vi "ConfigUI.vi"(8 "error in":errorcluster) -> (0 "error out":errorcluster)   [LabVIEW 2011]
uses:
  SubVIs/Controls/Control FP Objects - Operations.ctl
  SubVIs/Controls/INIT- READ - WRITE.ctl
  SubVIs/Controls/Init-Write-Read.ctl
  SubVIs/Controls/GetModueDescriptionsOperations.ctl
  SubVIs/Controls/Config UI Global Stop - Operations.ctl
  SubVIs/Controls/TransparencyEffectOperations.ctl
  SubVIs/Controls/ModulePicCluster.ctl
panel:
  in  "Stop":bool
  in  "Ready":bool
  in  "Testpanel":bool
  in  "Tab":enum32{"STATUS OK", "NO CHASSIS"}(tab)
  out "Info":string
  in  "BubbleTabs":T1(tab)
  in  "Slot BTN 8":bool
  in  "Slot BTN 7":bool
  in  "Slot BTN 6":bool
  in  "Slot BTN 5":bool
  in  "Slot BTN 4":bool
  in  "Slot BTN 3":bool
  in  "Slot BTN 2":bool
  in  "Slot BTN 1":bool
  out "ModSTR 8":string
  out "ModSTR 7":string
  out "ModSTR 6":string
  out "ModSTR 5":string
  out "ModSTR 4":string
  out "ModSTR 3":string
  out "ModSTR 2":string
  out "ModSTR 1":string
  out "Slot 8":picture
  out "Slot 7":picture
  out "Slot 6":picture
  out "Slot 5":picture
  out "Slot 4":picture
  out "Slot 3":picture
  out "Slot 2":picture
  out "Slot 1":picture
  out "CHASSIS_PIC":picture
  # "Configure your system by Clicking the modules"
  # "No CompactDAQ Chassis found! Please Connect your CompactDAQ Device or create simulated device in MAX!"
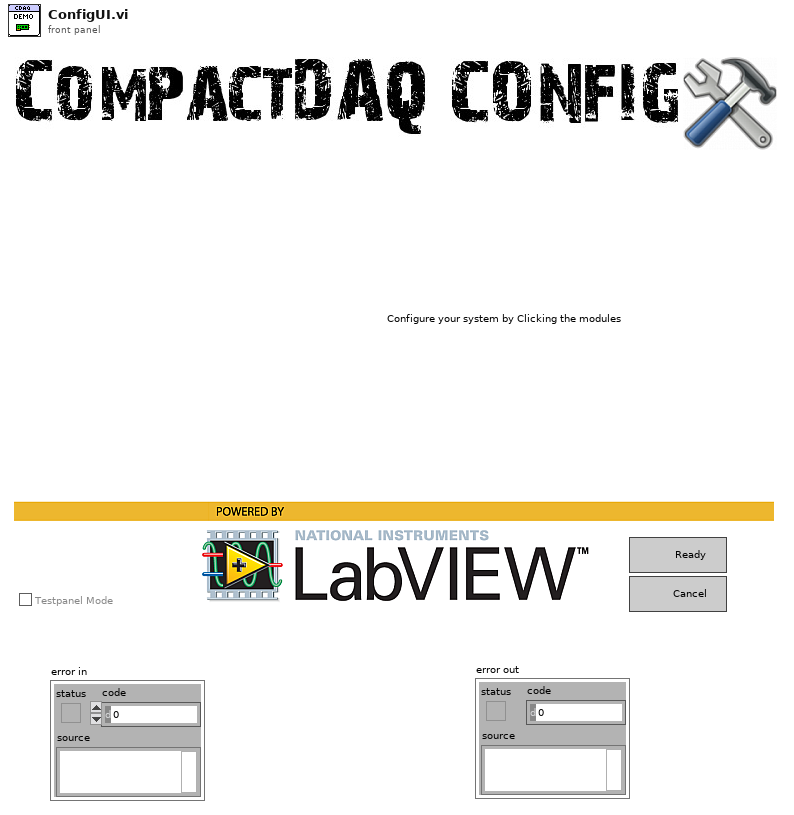
[diagram p1: front panel]
types:
  T1 = enum32{"Bubble1", "Bubble2", "Bubble3", "Bubble4", "Bubble5", "Bubble6", "Bubble7", "Bubble8", "EMPTY"}
  T2 = typedef "Control FP Objects - Operations.ctl" = enum16{"INIT", "CHANGE CHASSIS", "END"}
  T3 = typedef "INIT- READ - WRITE.ctl" = enum16{"INIT", "READ", "WRITE"}
  T4 = typedef "Init-Write-Read.ctl" = enum16{"INIT", "WRITE", "READ", "READ ALL"}
  T5 = typedef "GetModueDescriptionsOperations.ctl" = enum16{"INIT", "GET"}
  T6 = typedef "Config UI Global Stop - Operations.ctl" = enum16{"INIT", "STATUS", "STOP"}
  T7 = typedef "TransparencyEffectOperations.ctl" = enum16{"Show", "Hide 80%", "Hide All"}
  T8 = typedef "ModulePicCluster.ctl" = cluster{"Slot Nr":i32, "ModulePic":picture}
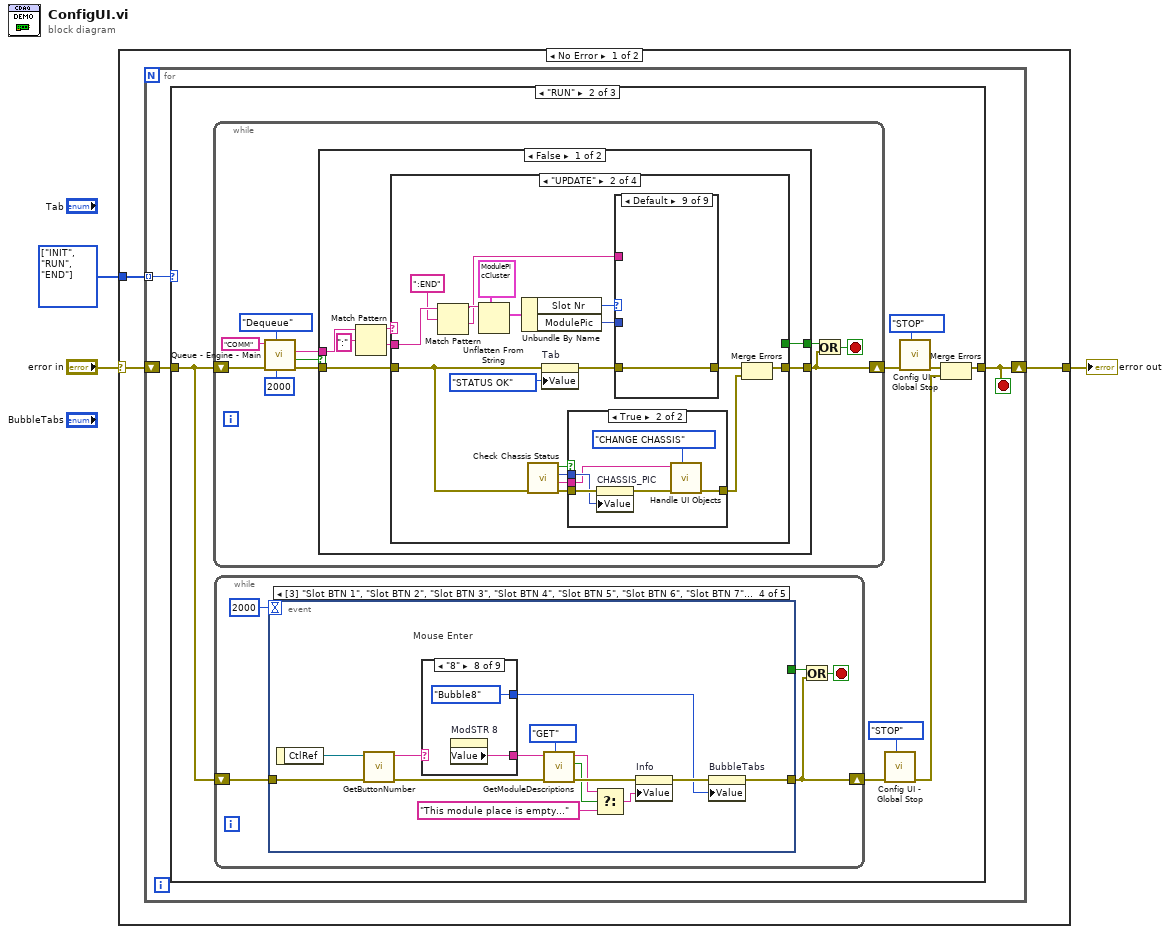
[diagram p0: block diagram]
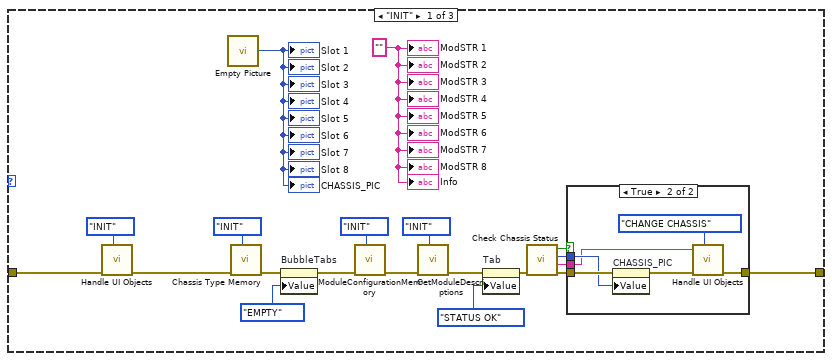
[diagram p2: hidden frame]
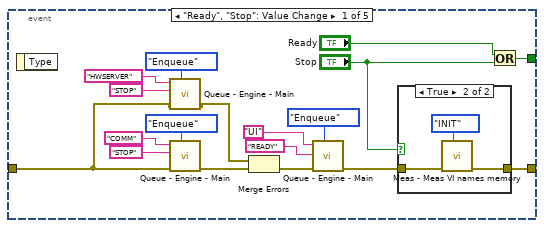
[diagram p4: hidden frame]
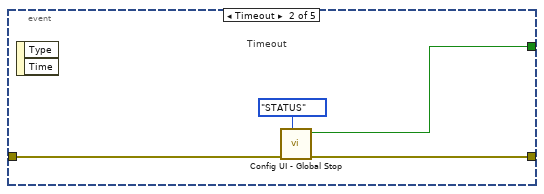
[diagram p6: hidden frame]
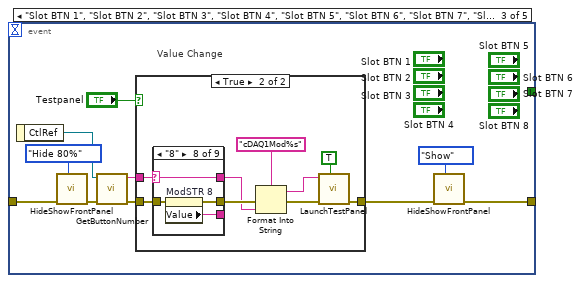
[diagram p7: hidden frame]
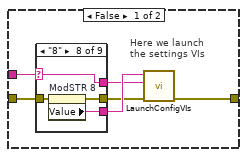
[diagram p8: hidden frame]
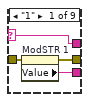
[diagram p9: hidden frame]
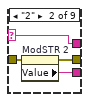
[diagram p10: hidden frame]
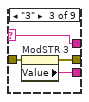
[diagram p11: hidden frame]
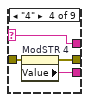
[diagram p12: hidden frame]
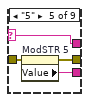
[diagram p13: hidden frame]
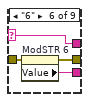
[diagram p14: hidden frame]
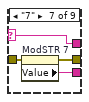
[diagram p15: hidden frame]
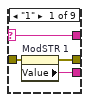
[diagram p17: hidden frame]
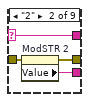
[diagram p18: hidden frame]
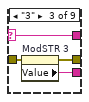
[diagram p19: hidden frame]
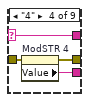
[diagram p20: hidden frame]
diagram:
  w3 = enum16{"INIT", "RUN", "END"}[] [enum."INIT", enum."RUN", enum."END"] items=["INIT", "RUN", "END"]
  n1 = case shown="No Error" "error in" {
    selector: "error in" -> [w4 w307]
    tunnel: w3 -> [w6 _]
    tunnel: [w5 w307] -> w2
    frame No Error {
      n2 = for {
        tunnel: w6 -> [w9] mode=indexing
        shift-right: [w7] -> w5
        shift-left: w4 -> [w8]
        stop <- w7 stop-if-true
        n3 = case shown="\"RUN\"" w9 {
          tunnel: [w18 w44 w303] -> w7
          tunnel: w8 -> [w13 w43 w306]
          frame "INIT" {
            w29 = "" ("ModSTR 1")
            n4 = call "Handle UI Objects.vi"("Operation"=Control_FP_Objects_-_Operations."INIT", "error in"=w13) -> ("error out"=w12:errorcluster)  [unwired: 9 in]
            n5 = call "Empty Picture"() -> ("empty picture"=→"Slot 1" →"Slot 2" →"Slot 3" →"Slot 4" →"Slot 5" →"Slot 6" →"Slot 7" →"Slot 8" →"CHASSIS_PIC":picture)
            n6 = call "Chassis Type Memory.vi"("Operation"=INIT-_READ_-_WRITE."INIT", "Error In"=w12) -> ("Error Out"=w15:errorcluster)  [unwired: 8 in, 1 out]
            n7 = property on="BubbleTabs" class="TabCtl (strict)"(error in=w15, "Value"=T1."EMPTY" ("BubbleTabs")) -> (error out=w14:errorcluster)  [unwired: 1 in, 1 out]
            n8 = call "ModuleConfigurationMemory.vi"("Operation"=Init-Write-Read."INIT", "Error In"=w14) -> ("Error Out"=w26:errorcluster)  [unwired: 5 in, 4 out]
            n9 = call "GetModuleDescriptions.vi"("Operation"=GetModueDescriptionsOperations."INIT", "Error In"=w26) -> ("Error Out"=w24:errorcluster)  [unwired: 7 in, 2 out]
            n10 = property on="Tab" class="TabCtl (strict)"(error in=w24, "Value"=enum32{"STATUS OK", "NO CHASSIS"}."STATUS OK" ("Tab")) -> (error out=w17:errorcluster)  [unwired: 1 in, 1 out]
            n11 = call "Check Chassis Status.vi"("error in (no error)"=w17) -> ("error out"=w21:errorcluster, "Chassis type Out"=w10:string, "Chassis Pic Out"=w20:picture, "Update?"=w19:bool)  [unwired: 7 in]
            n12 = case shown="True" w19 {
              tunnel: w21 -> [w30 w36]
              tunnel: [w30 w34] -> w18
              tunnel: w20 -> [_ w35]
              tunnel: w10 -> [_ w31]
              frame False {
                # "nothing to update"
              }
              frame True {
                n13 = property on="CHASSIS_PIC" class="Pict"(error in=w36, "Value"=w35) -> (error out=w33:errorcluster)  [unwired: 1 in, 1 out]
                n14 = call "Handle UI Objects.vi"("Operation"=Control_FP_Objects_-_Operations."CHANGE CHASSIS", "error in"=w33, "String In"=w31) -> ("error out"=w34:errorcluster)  [unwired: 8 in]
              }
            }
            "ModSTR 1" <- w29
            "ModSTR 2" <- w29
            "ModSTR 3" <- w29
            "ModSTR 4" <- w29
            "ModSTR 5" <- w29
            "ModSTR 7" <- w29
            "ModSTR 8" <- w29
            "ModSTR 6" <- w29
            "Info" <- w29
          }
          frame "RUN" {
            n15 = while {
              shift-right: [w214] -> w38
              shift-left: w43 -> [w208]
              stop <- w212 stop-if-true
              n16 = call "Queue - Engine - Main.vi"("timeout in ms (-1)"=2000, "Operation"=enum16{"Enqueue", "Dequeue", "Flush", "Release"}."Dequeue", "error in"=w208, "Queue Name In"="COMM" ("name (unnamed)")) -> ("error out"=w207:errorcluster, "timed out?"=w206:bool, "Data Out"=w205:string)  [unwired: 5 in]
              n17 = case shown="False" w206 {
                tunnel: w207 -> [w221 w290]
                tunnel: [w220 w288] -> w214
                tunnel: w205 -> [w218 _]
                tunnel: [w215 w287] -> w213
                frame False {
                  n18 = Match Pattern(string=w218, regular expression=":") -> (before substring=w219:string, after substring=w216:string)  [unwired: 1 in, 2 out]
                  n19 = case shown="\"UPDATE\"" w219 {
                    tunnel: w221 -> [w222 w230 w283 w285]
                    tunnel: [w222 w228 w282 w285] -> w220
                    tunnel: w216 -> [_ w234 _ _]
                    tunnel: [_ _ _ TRUE] -> w215
                    frame Default {
                    }
                    frame "UPDATE" {
                      n20 = Match Pattern(string=w234, regular expression=":END") -> (before substring=w236:string, after substring=w235:string)  [unwired: 1 in, 2 out]
                      n21 = Unflatten From String(type=T8 {"Slot Nr"=0, "ModulePic"=bytes[0]}, binary string=w236) -> (value=w239:T8)  [unwired: 3 in, 2 out]
                      n22 = Unbundle By Name(w239) -> ("Slot Nr"=w238:i32, "ModulePic"=w237:picture)
                      n23 = call "Check Chassis Status.vi"("error in (no error)"=w230) -> ("error out"=w227:errorcluster, "Chassis type Out"=w223:string, "Chassis Pic Out"=w225:picture, "Update?"=w224:bool)  [unwired: 7 in]
                      n24 = property on="Tab" class="TabCtl (strict)"(error in=w230, "Value"=enum32{"STATUS OK", "NO CHASSIS"}."STATUS OK" ("Tab")) -> (error out=w231:errorcluster)  [unwired: 1 in, 1 out]
                      n25 = case shown="True" w224 {
                        tunnel: w227 -> [w241 w247]
                        tunnel: [w241 w244] -> w226
                        tunnel: w225 -> [_ w246]
                        tunnel: w223 -> [_ w242]
                        frame False {
                          # "No update"
                        }
                        frame True {
                          n26 = property on="CHASSIS_PIC" class="Pict"(error in=w247, "Value"=w246) -> (error out=w245:errorcluster)  [unwired: 1 in, 1 out]
                          n27 = call "Handle UI Objects.vi"("Operation"=Control_FP_Objects_-_Operations."CHANGE CHASSIS", "error in"=w245, "String In"=w242) -> ("error out"=w244:errorcluster)  [unwired: 8 in]
                        }
                      }
                      n28 = case shown="Default" w238 {
                        tunnel: w237 -> [w249 w253 w257 w263 w267 w271 w275 w277 _]
                        tunnel: w231 -> [w251 w255 w259 w262 w266 w270 w274 w279 w280]
                        tunnel: [w250 w254 w258 w261 w265 w269 w273 w278 w280] -> w229
                        tunnel: w235 -> [w248 w252 w256 w260 w264 w268 w272 w276 _]
                        frame 1 {
                          n29 = property on="ModSTR 1" class="Str"("Value"=w248) -> ()  [unwired: 2 in, 2 out]
                          n30 = property on="Slot 1" class="Pict"(error in=w251, "Value"=w249) -> (error out=w250:errorcluster)  [unwired: 1 in, 1 out]
                        }
                        frame 2 {
                          n31 = property on="ModSTR 2" class="Str"("Value"=w252) -> ()  [unwired: 2 in, 2 out]
                          n32 = property on="Slot 2" class="Pict"(error in=w255, "Value"=w253) -> (error out=w254:errorcluster)  [unwired: 1 in, 1 out]
                        }
                        frame 3 {
                          n33 = property on="ModSTR 3" class="Str"("Value"=w256) -> ()  [unwired: 2 in, 2 out]
                          n34 = property on="Slot 3" class="Pict"(error in=w259, "Value"=w257) -> (error out=w258:errorcluster)  [unwired: 1 in, 1 out]
                        }
                        frame 4 {
                          n35 = property on="ModSTR 4" class="Str"("Value"=w260) -> ()  [unwired: 2 in, 2 out]
                          n36 = property on="Slot 4" class="Pict"(error in=w262, "Value"=w263) -> (error out=w261:errorcluster)  [unwired: 1 in, 1 out]
                        }
                        frame 5 {
                          n37 = property on="ModSTR 5" class="Str"("Value"=w264) -> ()  [unwired: 2 in, 2 out]
                          n38 = property on="Slot 5" class="Pict"(error in=w266, "Value"=w267) -> (error out=w265:errorcluster)  [unwired: 1 in, 1 out]
                        }
                        frame 6 {
                          n39 = property on="ModSTR 6" class="Str"("Value"=w268) -> ()  [unwired: 2 in, 2 out]
                          n40 = property on="Slot 6" class="Pict"(error in=w270, "Value"=w271) -> (error out=w269:errorcluster)  [unwired: 1 in, 1 out]
                        }
                        frame 7 {
                          n41 = property on="ModSTR 7" class="Str"("Value"=w272) -> ()  [unwired: 2 in, 2 out]
                          n42 = property on="Slot 7" class="Pict"(error in=w274, "Value"=w275) -> (error out=w273:errorcluster)  [unwired: 1 in, 1 out]
                        }
                        frame 8 {
                          n43 = property on="ModSTR 8" class="Str"("Value"=w276) -> ()  [unwired: 2 in, 2 out]
                          n44 = property on="Slot 8" class="Pict"(error in=w279, "Value"=w277) -> (error out=w278:errorcluster)  [unwired: 1 in, 1 out]
                        }
                        frame Default {
                        }
                      }
                      n45 = Merge Errors(w229, w226) -> (w228:errorcluster)
                    }
                    frame "NO CHASSIS" {
                      n46 = property on="Tab" class="TabCtl (strict)"(error in=w283, "Value"=enum32{"STATUS OK", "NO CHASSIS"}."NO CHASSIS" ("Tab")) -> (error out=w282:errorcluster)  [unwired: 1 in, 1 out]
                    }
                    frame "STOP" {
                    }
                  }
                }
                frame True {
                  # "Timeout"
                  n47 = call "Check Chassis Status.vi"("error in (no error)"=w290) -> ("error out"=w294:errorcluster, "Chassis type Out"=w291:string, "Chassis Pic Out"=w293:picture, "Update?"=w292:bool)  [unwired: 7 in]
                  n48 = case shown="True" w292 {
                    tunnel: w294 -> [w295 w301]
                    tunnel: [w295 w298] -> w289
                    tunnel: w293 -> [_ w300]
                    tunnel: w291 -> [_ w297]
                    frame False {
                    }
                    frame True {
                      n49 = property on="CHASSIS_PIC" class="Pict"(error in=w301, "Value"=w300) -> (error out=w299:errorcluster)  [unwired: 1 in, 1 out]
                      n50 = call "Handle UI Objects.vi"("Operation"=Control_FP_Objects_-_Operations."CHANGE CHASSIS", "error in"=w299, "String In"=w297) -> ("error out"=w298:errorcluster)  [unwired: 8 in]
                    }
                  }
                  n51 = call "Config UI - Global Stop.vi"("Operation"=Config_UI_Global_Stop_-_Operations."STATUS", "error in (no error)"=w289) -> ("error out"=w288:errorcluster, "Stop?"=w287:bool)  [unwired: 8 in]
                }
              }
              n52 = Or(x=w213, y=w214) -> (x .or. y?=w212:bool)
            }
            n53 = while {
              shift-right: [w48] -> w42
              shift-left: w43 -> [w49]
              stop <- w46 stop-if-true
              n54 = event shown="[3] \"Slot BTN 1\", \"Slot BTN 2\", \"Slot BTN 3\", \"Slot BTN 4\", \"Slot BTN 5\", \"Slot BTN 6\", \"Slot BTN 7\", \"Slot BTN 8\": Mouse Enter" {
                selector: _ -> [_ _ _ _ _]
                dyn-events: _ -> [_ _ _ _ _]
                timeout: 2000 -> [_ _ _ _ _]
                tunnel: [w53 w74 _ _ _] -> w47
                tunnel: [w50 w72 w78 w174 w201] -> w48
                tunnel: w49 -> [w60 w73 w81 w181 w203]
                event "Ready", "Stop": Value Change {
                  n55 = event-data() -> ()  [unwired: 1 in, 1 out]
                  n56 = call "Queue - Engine - Main.vi"("Operation"=enum16{"Enqueue", "Dequeue", "Flush", "Release"}."Enqueue", "error in"=w60, "Queue Data In"="STOP" ("element"), "Queue Name In"="HWSERVER" ("name (unnamed)")) -> ("error out"=w59:errorcluster)  [unwired: 5 in, 2 out]
                  n57 = call "Queue - Engine - Main.vi"("Operation"=enum16{"Enqueue", "Dequeue", "Flush", "Release"}."Enqueue", "error in"=w60, "Queue Data In"="STOP" ("element"), "Queue Name In"="COMM" ("name (unnamed)")) -> ("error out"=w65:errorcluster)  [unwired: 5 in, 2 out]
                  n58 = Merge Errors(w59, w65) -> (w55:errorcluster)
                  n59 = call "Queue - Engine - Main.vi"("Operation"=enum16{"Enqueue", "Dequeue", "Flush", "Release"}."Enqueue", "error in"=w55, "Queue Data In"="READY" ("Queue Name In"), "Queue Name In"="UI") -> ("error out"=w51:errorcluster)  [unwired: 5 in, 2 out]
                  n60 = case shown="True" "Stop" {
                    tunnel: w51 -> [w68 w69]
                    tunnel: [w68 w70] -> w50
                    frame False {
                    }
                    frame True {
                      n61 = call "Meas - Meas VI names memory.vi"("Operation"=INIT-_READ_-_WRITE."INIT", "Error In"=w69) -> ("Error Out"=w70:errorcluster)  [unwired: 8 in, 1 out]
                    }
                  }
                  n62 = Or(x="Ready", y="Stop") -> (x .or. y?=w53:bool)
                }
                event Timeout {
                  # "Timeout"
                  n63 = event-data() -> ()  [unwired: 1 in, 2 out]
                  n64 = call "Config UI - Global Stop.vi"("Operation"=Config_UI_Global_Stop_-_Operations."STATUS", "error in (no error)"=w73) -> ("error out"=w72:errorcluster, "Stop?"=w74:bool)  [unwired: 8 in]
                }
                event "Slot BTN 1", "Slot BTN 2", "Slot BTN 3", "Slot BTN 4", "Slot BTN 5", "Slot BTN 6", "Slot BTN 7", "Slot BTN 8": Value Change {
                  # "Value Change"
                  n65 = event-data() -> ("CtlRef"=w85:refnum<vi>)  [unwired: 1 in]
                  n66 = call "HideShowFrontPanel.vi"("Operation"=TransparencyEffectOperations."Hide 80%", "Error In"=w81) -> ("Error Out"=w80:errorcluster)  [unwired: 9 in]
                  n67 = call "GetButtonNumber.vi"("Error In"=w80, "BTN Ref In"=w85) -> ("Error Out"=w83:errorcluster, "BTN Nr Out"=w84:string)  [unwired: 8 in]
                  n68 = case shown="True" "Testpanel" {
                    tunnel: [w86 w134] -> w76
                    tunnel: w84 -> [w90 w128]
                    tunnel: w83 -> [w89 w130]
                    frame False {
                      # "Here we launch\nthe settings VIs"
                      n69 = case shown="\"8\"" w90 {
                        selector: w90 -> [w92 w96 w100 w104 w108 w112 w116 w120 w124]
                        tunnel: [w95 w99 w103 w107 w111 w115 w119 w123 _] -> w91
                        tunnel: w89 -> [w94 w98 w102 w106 w110 w114 w118 w122 w125]
                        tunnel: [w93 w97 w101 w105 w109 w113 w117 w121 w125] -> w88
                        tunnel: [w92 w96 w100 w104 w108 w112 w116 w120 w124] -> w87
                        frame "1" {
                          n70 = property on="ModSTR 1" class="Str"(error in=w94) -> (error out=w93:errorcluster, "Value"=w95:string)  [unwired: 1 in, 1 out]
                        }
                        frame "2" {
                          n71 = property on="ModSTR 2" class="Str"(error in=w98) -> (error out=w97:errorcluster, "Value"=w99:string)  [unwired: 1 in, 1 out]
                        }
                        frame "3" {
                          n72 = property on="ModSTR 3" class="Str"(error in=w102) -> (error out=w101:errorcluster, "Value"=w103:string)  [unwired: 1 in, 1 out]
                        }
                        frame "4" {
                          n73 = property on="ModSTR 4" class="Str"(error in=w106) -> (error out=w105:errorcluster, "Value"=w107:string)  [unwired: 1 in, 1 out]
                        }
                        frame "5" {
                          n74 = property on="ModSTR 5" class="Str"(error in=w110) -> (error out=w109:errorcluster, "Value"=w111:string)  [unwired: 1 in, 1 out]
                        }
                        frame "6" {
                          n75 = property on="ModSTR 6" class="Str"(error in=w114) -> (error out=w113:errorcluster, "Value"=w115:string)  [unwired: 1 in, 1 out]
                        }
                        frame "7" {
                          n76 = property on="ModSTR 7" class="Str"(error in=w118) -> (error out=w117:errorcluster, "Value"=w119:string)  [unwired: 1 in, 1 out]
                        }
                        frame "8" {
                          n77 = property on="ModSTR 8" class="Str"(error in=w122) -> (error out=w121:errorcluster, "Value"=w123:string)  [unwired: 1 in, 1 out]
                        }
                        frame Default {
                        }
                      }
                      n78 = call "LaunchConfigVIs.vi"("Error In"=w88, "Device Name"=w87, "Module Name"=w91) -> ("Error Out"=w86:errorcluster)  [unwired: 8 in]
                    }
                    frame True {
                      n79 = case shown="\"8\"" w128 {
                        selector: w128 -> [w135 w139 w143 w147 w151 w155 w159 w163 w167]
                        tunnel: [w138 w142 w146 w150 w154 w158 w162 w166 _] -> _
                        tunnel: w130 -> [w137 w141 w145 w149 w153 w157 w161 w165 w168]
                        tunnel: [w136 w140 w144 w148 w152 w156 w160 w164 w168] -> w129
                        tunnel: [w135 w139 w143 w147 w151 w155 w159 w163 w167] -> w127
                        frame "1" {
                          n80 = property on="ModSTR 1" class="Str"(error in=w137) -> (error out=w136:errorcluster, "Value"=w138:string)  [unwired: 1 in, 1 out]
                        }
                        frame "2" {
                          n81 = property on="ModSTR 2" class="Str"(error in=w141) -> (error out=w140:errorcluster, "Value"=w142:string)  [unwired: 1 in, 1 out]
                        }
                        frame "3" {
                          n82 = property on="ModSTR 3" class="Str"(error in=w145) -> (error out=w144:errorcluster, "Value"=w146:string)  [unwired: 1 in, 1 out]
                        }
                        frame "4" {
                          n83 = property on="ModSTR 4" class="Str"(error in=w149) -> (error out=w148:errorcluster, "Value"=w150:string)  [unwired: 1 in, 1 out]
                        }
                        frame "5" {
                          n84 = property on="ModSTR 5" class="Str"(error in=w153) -> (error out=w152:errorcluster, "Value"=w154:string)  [unwired: 1 in, 1 out]
                        }
                        frame "6" {
                          n85 = property on="ModSTR 6" class="Str"(error in=w157) -> (error out=w156:errorcluster, "Value"=w158:string)  [unwired: 1 in, 1 out]
                        }
                        frame "7" {
                          n86 = property on="ModSTR 7" class="Str"(error in=w161) -> (error out=w160:errorcluster, "Value"=w162:string)  [unwired: 1 in, 1 out]
                        }
                        frame "8" {
                          n87 = property on="ModSTR 8" class="Str"(error in=w165) -> (error out=w164:errorcluster, "Value"=w166:string)  [unwired: 1 in, 1 out]
                        }
                        frame Default {
                        }
                      }
                      n88 = Format Into String(format string="cDAQ1Mod%s", error in=w129, w127) -> (resulting string=w132:string, error out=w126:errorcluster)  [unwired: 1 in]
                      n89 = call "LaunchTestPanel.vi"("Wait Until Completion (T)?"=TRUE, "Error In"=w126, "Device name In"=w132) -> ("Error Out"=w134:errorcluster)  [unwired: 8 in]
                    }
                  }
                  n90 = call "HideShowFrontPanel.vi"("Operation"=TransparencyEffectOperations."Show", "Error In"=w76) -> ("Error Out"=w78:errorcluster)  [unwired: 9 in]
                }
                event "Slot BTN 1", "Slot BTN 2", "Slot BTN 3", "Slot BTN 4", "Slot BTN 5", "Slot BTN 6", "Slot BTN 7", "Slot BTN 8": Mouse Enter {
                  # "Mouse Enter"
                  n91 = event-data() -> ("CtlRef"=w182:refnum<vi>)  [unwired: 1 in]
                  n92 = call "GetButtonNumber.vi"("Error In"=w181, "BTN Ref In"=w182) -> ("Error Out"=w179:errorcluster, "BTN Nr Out"=w177:string)  [unwired: 8 in]
                  n93 = case shown="\"8\"" w177 {
                    tunnel: [w184 w186 w188 w190 w192 w194 w196 w198 _] -> w176
                    tunnel: [T1."Bubble1" ("BubbleTabs") T1."Bubble2" ("BubbleTabs") T1."Bubble3" ("BubbleTabs") T1."Bubble4" ("BubbleTabs") T1."Bubble5" ("BubbleTabs") T1."Bubble6" ("BubbleTabs") T1."Bubble7" ("BubbleTabs") T1."Bubble8" ("BubbleTabs") T1."EMPTY" ("BubbleTabs")] -> w173
                    frame "1" {
                      n94 = property on="ModSTR 1" class="Str"() -> ("Value"=w184:string)  [unwired: 2 in, 2 out]
                    }
                    frame "2" {
                      n95 = property on="ModSTR 2" class="Str"() -> ("Value"=w186:string)  [unwired: 2 in, 2 out]
                    }
                    frame "3" {
                      n96 = property on="ModSTR 3" class="Str"() -> ("Value"=w188:string)  [unwired: 2 in, 2 out]
                    }
                    frame "4" {
                      n97 = property on="ModSTR 4" class="Str"() -> ("Value"=w190:string)  [unwired: 2 in, 2 out]
                    }
                    frame "5" {
                      n98 = property on="ModSTR 5" class="Str"() -> ("Value"=w192:string)  [unwired: 2 in, 2 out]
                    }
                    frame "6" {
                      n99 = property on="ModSTR 6" class="Str"() -> ("Value"=w194:string)  [unwired: 2 in, 2 out]
                    }
                    frame "7" {
                      n100 = property on="ModSTR 7" class="Str"() -> ("Value"=w196:string)  [unwired: 2 in, 2 out]
                    }
                    frame "8" {
                      n101 = property on="ModSTR 8" class="Str"() -> ("Value"=w198:string)  [unwired: 2 in, 2 out]
                    }
                    frame Default {
                    }
                  }
                  n102 = call "GetModuleDescriptions.vi"("Operation"=GetModueDescriptionsOperations."GET", "Error In"=w179, "Module Name In"=w176) -> ("Error Out"=w178:errorcluster, "Found?"=w172:bool, "Data Out"=w171:string)  [unwired: 6 in]
                  n103 = Select(t=w171, s=w172, f="This module place is empty...") -> (s? t:f=w169:string)
                  n104 = property on="Info" class="Str"(error in=w178, "Value"=w169) -> (error out=w175:errorcluster)  [unwired: 1 in, 1 out]
                  n105 = property on="BubbleTabs" class="TabCtl (strict)"(error in=w175, "Value"=w173) -> (error out=w174:errorcluster)  [unwired: 1 in, 1 out]
                }
                event "Slot BTN 1", "Slot BTN 2", "Slot BTN 3", "Slot BTN 4", "Slot BTN 5", "Slot BTN 6", "Slot BTN 7", "Slot BTN 8": Mouse Leave {
                  # "Mouse leave"
                  n106 = event-data() -> ()  [unwired: 1 in, 1 out]
                  n107 = property on="Info" class="Str"(error in=w203, "Value"="" ("Info")) -> (error out=w202:errorcluster)  [unwired: 1 in, 1 out]
                  n108 = property on="BubbleTabs" class="TabCtl (strict)"(error in=w202, "Value"=T1."EMPTY" ("BubbleTabs")) -> (error out=w201:errorcluster)  [unwired: 1 in, 1 out]
                }
              }
              n109 = Or(x=w47, y=w48) -> (x .or. y?=w46:bool)
            }
            n110 = call "Config UI - Global Stop.vi"("Operation"=Config_UI_Global_Stop_-_Operations."STOP", "error in (no error)"=w42) -> ("error out"=w41:errorcluster)  [unwired: 8 in, 1 out]
            n111 = call "Config UI - Global Stop.vi"("Operation"=Config_UI_Global_Stop_-_Operations."STOP", "error in (no error)"=w38) -> ("error out"=w37:errorcluster)  [unwired: 8 in, 1 out]
            n112 = Merge Errors(w37, w41) -> (w44:errorcluster)
          }
          frame "END" {
            n113 = control-ref of="This VI"() -> (w302:refnum<vi>)
            n114 = call "TransparencyEffect.vi"("Operation"=TransparencyEffectOperations."Hide All", "error in"=w306, "VI Ref in"=w302) -> ("error out"=w304:errorcluster)  [unwired: 8 in]
            n115 = invoke class="VI" method="FP.Close"(reference=w302, error in=w304) -> (error out=w303:errorcluster)  [unwired: 1 in, 2 out]
          }
        }
      }
    }
    frame Error {
    }
  }
  "error out" <- w2
